vi "Write On Timeout Status.vi"(8 "error in (no error)":errorcluster, 10 "On Count Status":T1, 11 "Repeat Until Timeout in":refnum<class "bt_Repeat Until Timeout.lvclass">) -> (0 "error out":errorcluster, 3 "Repeat Until Timeout out":refnum<class "bt_Repeat Until Timeout.lvclass">)   [LabVIEW 2021, in "BT.lvlib" / "bt_Repeat Until Timeout.lvclass"]
uses:
  bt_Repeat Until Timeout.lvclass
  Support/On Timeout Status - Type.ctl
  bt_Repeat Until Timeout.lvclass/bt_Repeat Until Timeout.ctl
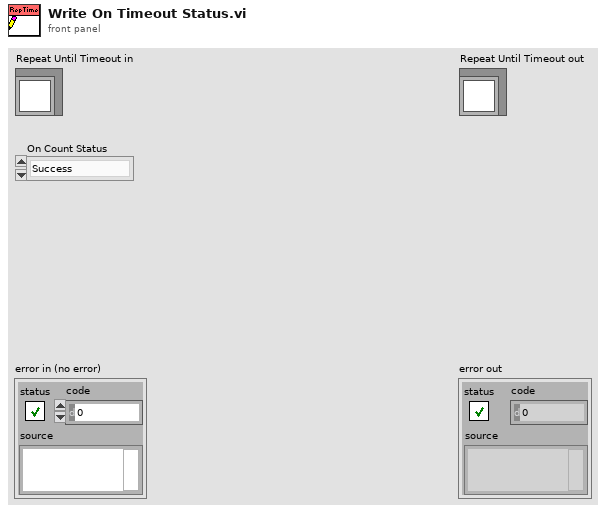
[diagram p1: front panel]
types:
  T1 = typedef "BT.lvlib/bt_Repeat Until Timeout.lvclass/On Timeout Status - Type.ctl" = enum16{"Success", "Failure"}
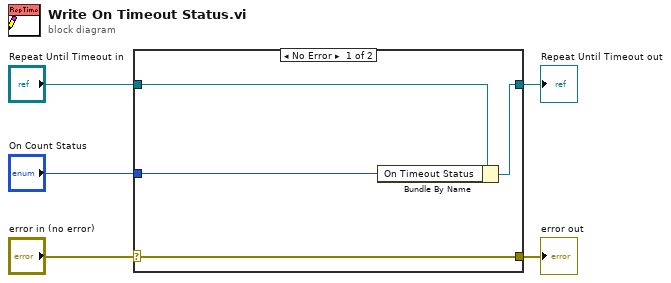
[diagram p0: block diagram]
diagram:
  n1 = case shown="No Error" "error in (no error)" {
    selector: "error in (no error)" -> [w9 w10]
    tunnel: [w9 w10] -> w4
    tunnel: [w7 w11] -> w2
    tunnel: "Repeat Until Timeout in" -> [w8 w11]
    tunnel: "On Count Status" -> [w6 _]
    frame No Error {
      n2 = Bundle By Name(cluster=w8, "On Timeout Status"=w6) -> (w7:refnum<class "bt_Repeat Until Timeout.lvclass">)
    }
    frame Error {
    }
  }
  "error out" <- w4
  "Repeat Until Timeout out" <- w2
